vi "runner.vi"() -> ()   [LabVIEW 2010]
uses:
  common/xcontrols/XUserDropdown/XUserDropdown/XUserDropdown.xctl
  common/classes/ErrorController/ErrorController/ErrorController.lvclass
  <vilib>/Utility/miscctls.llb/LVPointTypeDef.ctl
  common/clusters/plugin_specification.ctl
  HelioWizardDL101109/wizard_cluster.ctl
  common/classes/GenericComponent/GenericComponent/GenericComponent.lvclass
  <vilib>/Platform/browser.llb/Open URL in Default Browser (string).vi
  common/classes/ErrorController/ErrorController/class_data.vi
panel:
  out "error loaded?":bool
  out "progress slider":i32(slide) scale=0.0..13.0
  in  "button: copy user":bool
  in  "button: delete user":bool
  in  "button: new user":bool
  in  "user":string(xcontrol)
  in  "mainConfigButton":bool
  in  "step":i32(listbox) caption="steps"
  in  "proceedButton":bool
  in  "backButton":bool
  in  "startButton":bool
  in  "wizard":string(combo) caption="Select a wizard"
  # "Wizard Runner"
  # "Procedure\n\n1. Select and start a wizard (it may take some time until all steps are loaded).\n\n2. Perform all configuration steps in the sequence given (note that there may be dependencies!).\n\n3. Edit main configuration.\n\nHint: Don't leave any component specifications empty in the configuration dialogs. Choose the generic version if a more specifiy component doesn't apply."
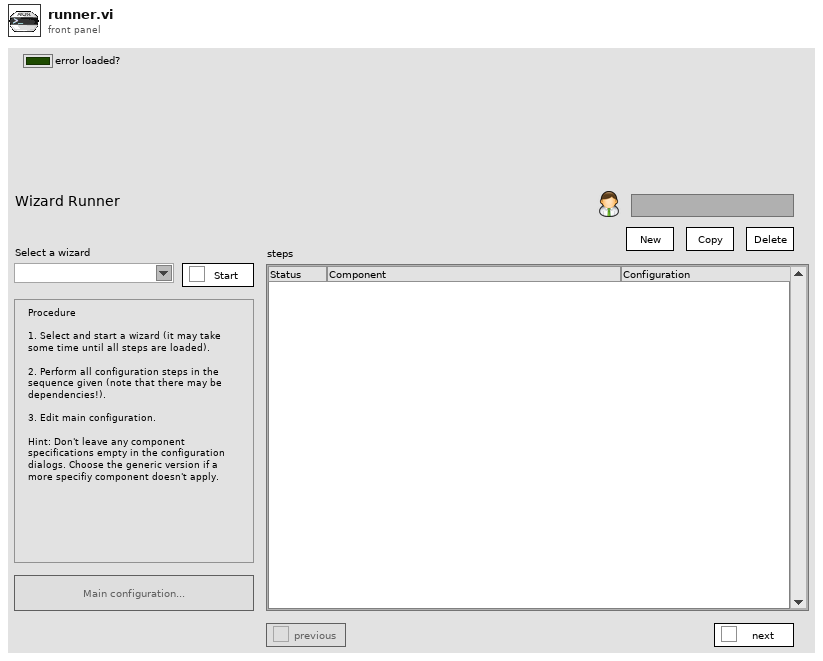
[diagram p1: front panel]
types:
  T1 = typedef "LVPointTypeDef.ctl" = cluster{"Horizontal":i16, "Vertical":i16}
  T2 = typedef "plugin_specification.ctl" = cluster{"class path":string, "configuration":string, "label":string, "settings name":string}
  T3 = typedef "wizard_cluster.ctl" = cluster{"step":T2[]}
  T4 = enum8{"Enabled", "Disabled", "Disabled and Grayed Out"}
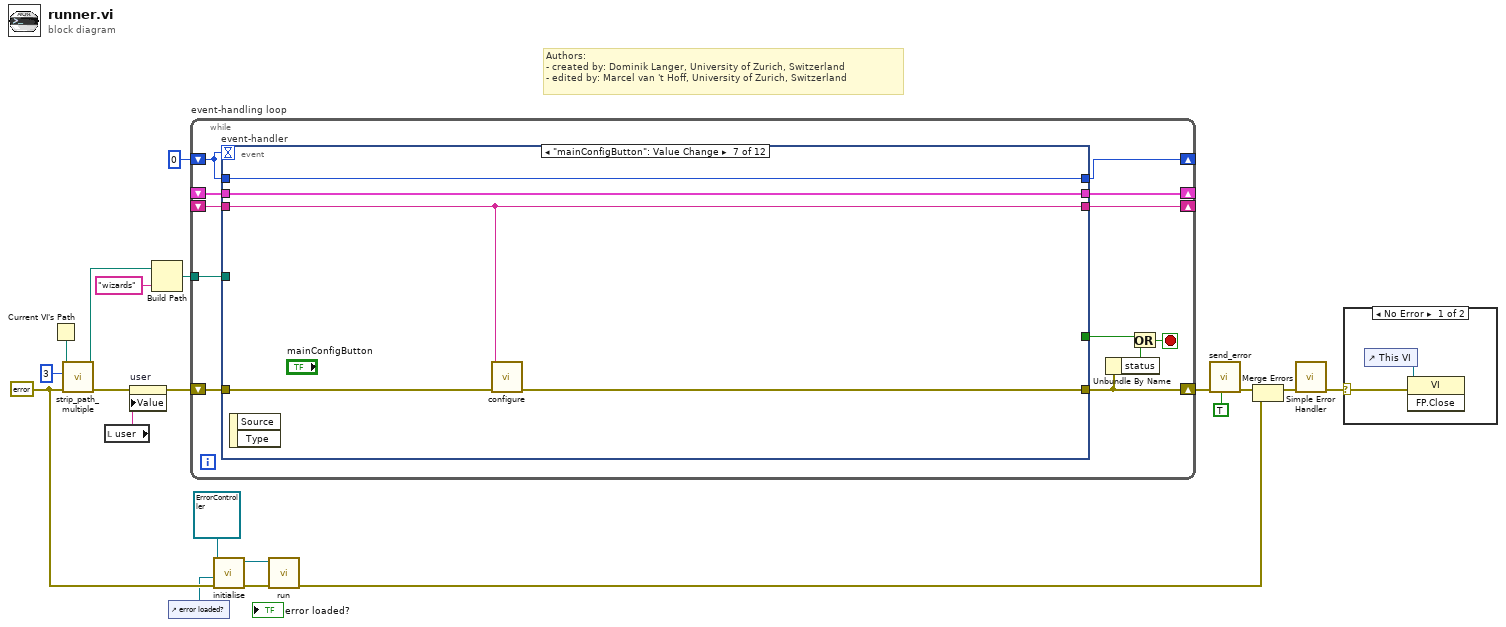
[diagram p0: block diagram]
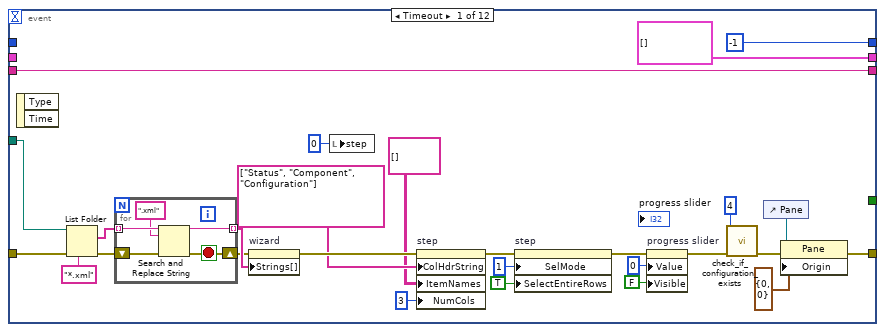
[diagram p3: hidden frame]
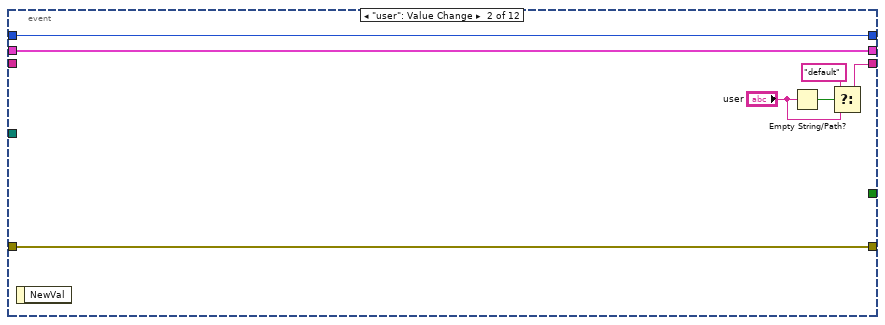
[diagram p4: hidden frame]
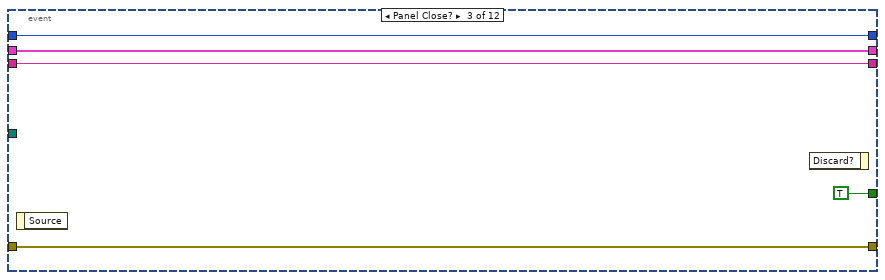
[diagram p5: hidden frame]
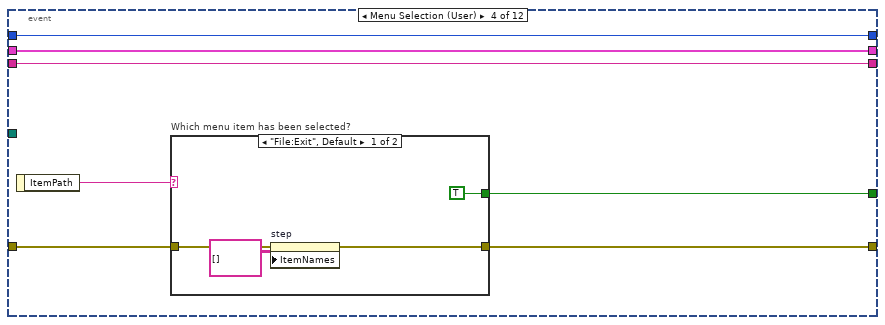
[diagram p6: hidden frame]
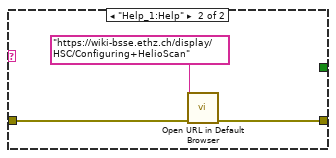
[diagram p7: hidden frame]
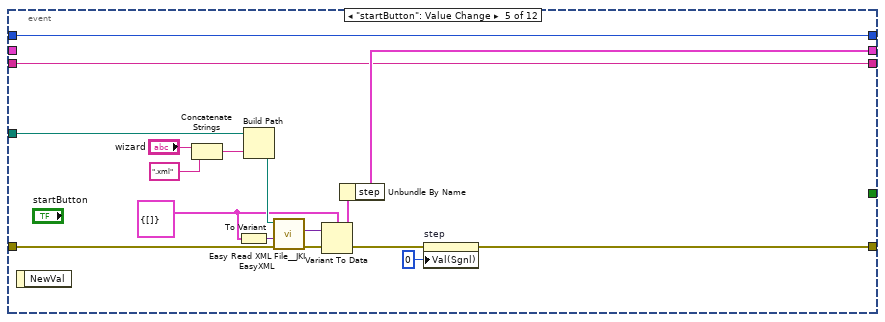
[diagram p8: hidden frame]
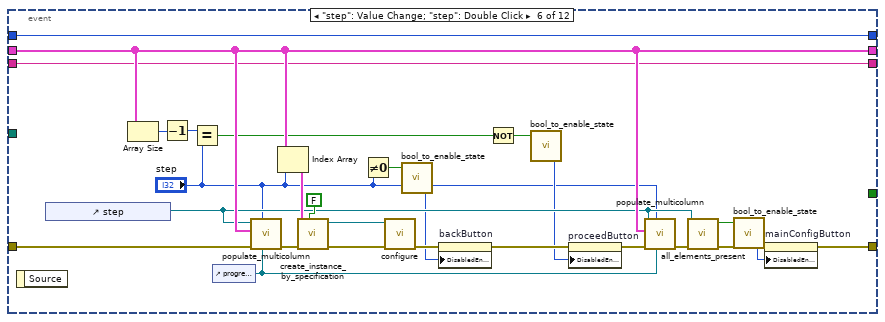
[diagram p9: hidden frame]
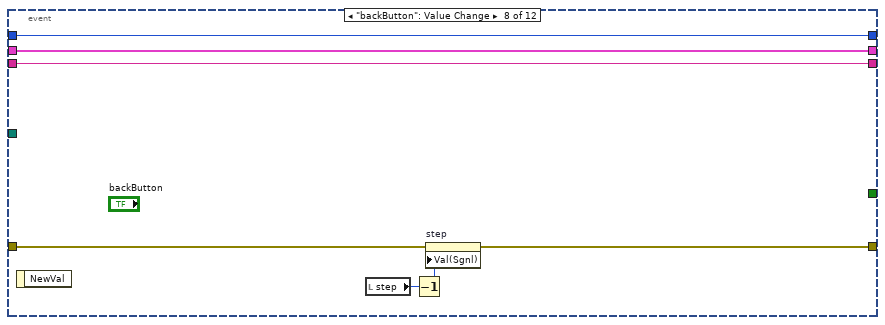
[diagram p10: hidden frame]
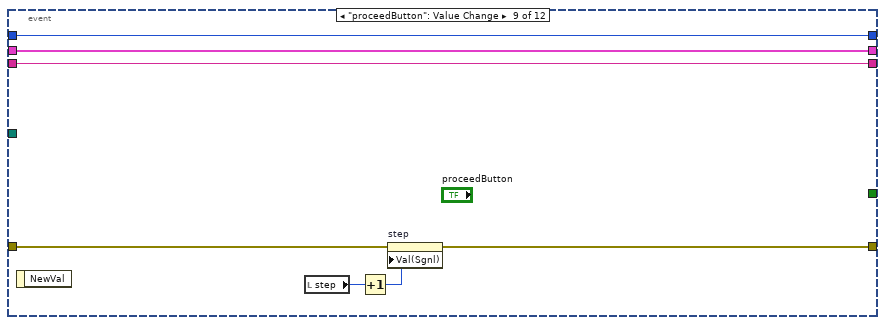
[diagram p11: hidden frame]
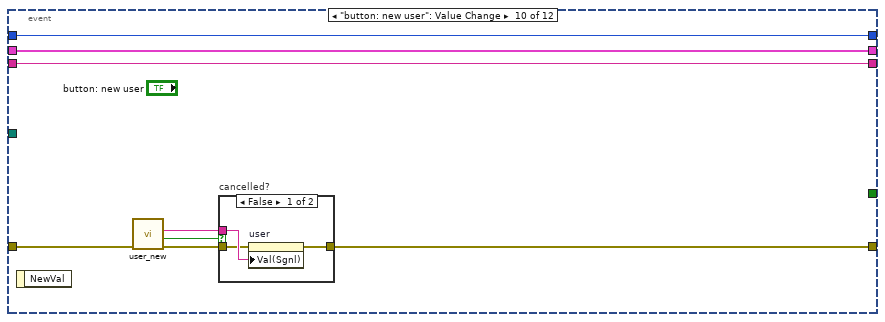
[diagram p12: hidden frame]
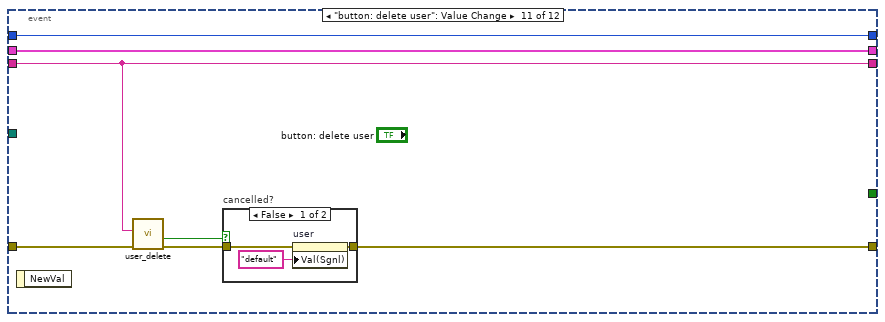
[diagram p14: hidden frame]
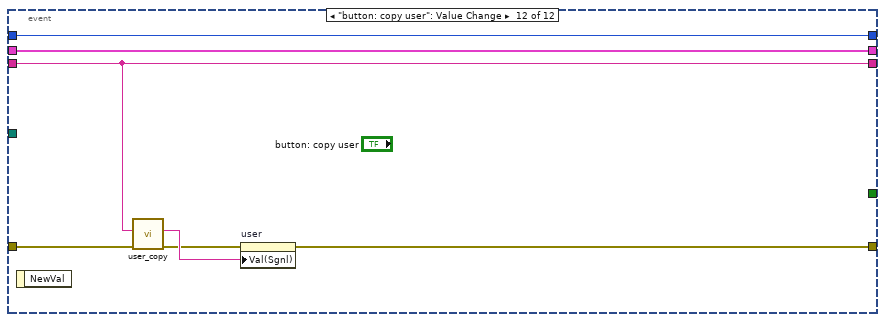
[diagram p16: hidden frame]
diagram:
  w5 = errorcluster {"status"=FALSE, "code"=0, "source"=""} ("error in (no error)")
  # "Authors: \n- created by: Dominik Langer, University of Zurich, Switzerland\n- edited by: Marcel van 't Hoff, University of Zurich, Switzerland"
  n1 = Current VI's Path() -> (path=w17:path)
  n2 = call "strip_path_multiple.vi"("error in (no error)"=w5, "number of strips"=3, "path in"=w17) -> ("error out"=w3:errorcluster, "path out"=w16:path)  [unwired: 7 in]
  n3 = local read "user"() -> (w1:string)
  n4 = property on="user" class="XUserDropdown (strict)"(error in=w3, "Value"=w1) -> (error out=w2:errorcluster)  [unwired: 1 in, 1 out]
  n5 = Build Path(base path=w16, name or relative path="wizards") -> (appended path=w18:path)
  n6 = control-ref of="error loaded?"() -> (w4:refnum<vi>)
  n7 = while "event-handling loop" {
    tunnel: w18 -> [w27]
    shift-right: [w25] -> _
    shift-left: _ -> [w26]
    shift-right: [w23] -> _
    shift-left: 0 -> [w24]
    shift-right: [w22] -> _
    shift-left: _ -> [w21]
    shift-right: [w31] -> w10
    shift-left: w2 -> [w32]
    stop <- w28 stop-if-true
    n8 = event "event-handler" shown="[6] \"mainConfigButton\": Value Change" {
      selector: _ -> [_ _ _ _ _ _ _ _ _ _ _ _]
      dyn-events: _ -> [_ _ _ _ _ _ _ _ _ _ _ _]
      timeout: w24 -> [_ _ _ _ _ _ _ _ _ _ _ _]
      tunnel: w32 -> [w56 w69 w76 w79 w107 w127 w137 w141 w149 w158 w170 w181]
      tunnel: [w35 w69 w76 w78 w95 w120 w136 w144 w148 w155 w167 w177] -> w31
      tunnel: [_ _ TRUE w80 _ _ _ _ _ _ _ _] -> w29
      tunnel: w27 -> [w57 _ _ _ w106 _ _ _ _ _ _ _]
      tunnel: [T2[] [] w71 w74 w83 w98 w124 w139 w146 w153 w161 w172 w183] -> w25
      tunnel: w26 -> [_ w71 w74 w83 _ w124 w139 w146 w153 w161 w172 w183]
      tunnel: [-1 w70 w73 w82 w101 w129 w138 w145 w152 w160 w171 w182] -> w23
      tunnel: w24 -> [_ w70 w73 w82 w101 w129 w138 w145 w152 w160 w171 w182]
      tunnel: [w46 w66 w72 w77 w94 w119 w135 w140 w147 w159 w169 w180] -> w22
      tunnel: w21 -> [w46 _ w72 w77 w94 w119 w135 w140 w147 w159 w169 w180]
      event Timeout {
        n9 = event-data() -> ()  [unwired: 1 in, 2 out]
        n10 = List Folder(path=w57, pattern="*.xml", error in=w56) -> (filenames=w40:string[], error out=w38:errorcluster)  [unwired: 1 in, 2 out]
        n11 = for {
          tunnel: w40 -> [w64] mode=indexing
          tunnel: [w62] -> w39 mode=indexing
          shift-right: [w60] -> w37
          shift-left: w38 -> [w61]
          stop <- w60 stop-if-true
          n12 = Search and Replace String(input string=w64, search string=".xml", error in=w61) -> (result string=w62:string, error out=w60:errorcluster)  [unwired: 5 in, 2 out]
        }
        n13 = property on="wizard" class="CmbBox"(error in=w37, "Strings[]"=w39) -> (error out=w54:errorcluster)  [unwired: 1 in, 1 out]
        n14 = local write "step"(0 ("step")) -> ()
        n15 = property on="step" class="MCListbox (strict)"(error in=w54, "ColHdrString"=string[] ["Status", "Component", "Configuration"] ("Item Names"), "ItemNames"=string[][] [] ("Item Names"), "NumCols"=u32 3 ("Number of Columns")) -> (error out=w48:errorcluster)  [unwired: 1 in, 1 out]
        n16 = property on="step" class="MCListbox (strict)"(error in=w48, "SelMode"=1 ("Selection Mode"), "SelectEntireRows"=TRUE ("Select Entire Rows")) -> (error out=w43:errorcluster)  [unwired: 1 in, 1 out]
        n17 = property on="progress slider" class="Slide (strict)"(error in=w43, "Value"=0 ("progress slider"), "Visible"=FALSE) -> (error out=w42:errorcluster)  [unwired: 1 in, 1 out]
        n18 = call "check_if_configuration_exists.vi"("error in (no error)"=w42, "number of strips"=4) -> ("error out"=w36:errorcluster)  [unwired: 9 in]
        n19 = control-ref of="Pane"() -> (w34:refnum<vi>)
        n20 = property class="Pane"(reference=w34, error in=w36, "Origin"=T1 {"Horizontal"=0, "Vertical"=0}) -> (error out=w35:errorcluster)  [unwired: 1 out]
      }
      event "user": Value Change {
        n21 = event-data() -> ()  [unwired: 1 in, 1 out]
        n22 = Empty String/Path?(string/path="user") -> (empty?=w68:bool)
        n23 = Select(t="default", s=w68, f="user") -> (s? t:f=w66:string)
      }
      event Panel Close? {
        n24 = event-data() -> ()  [unwired: 1 in, 1 out]
        n25 = event-data() -> ()  [unwired: 2 in, 1 out]
      }
      event Menu Selection (User) {
        n26 = event-data() -> ("ItemPath"=w81:string)  [unwired: 1 in]
        n27 = case "Which menu item has been selected?" shown="\"File:Exit\", Default" w81 {
          tunnel: [TRUE _] -> w80
          tunnel: w79 -> [w86 w90]
          tunnel: [w84 w89] -> w78
          frame "File:Exit", Default {
            n28 = property on="step" class="MCListbox (strict)"(error in=w86, "ItemNames"=string[][] [] ("Item Names")) -> (error out=w84:errorcluster)  [unwired: 1 in, 1 out]
          }
          frame "Help_1:Help" {
            n29 = call-poly <vilib>:"Open URL in Default Browser.vi"("error in (no error)"=w90, "URL"="https://wiki-bsse.ethz.ch/display/HSC/Configuring+HelioScan") -> ("error out"=w89:errorcluster)  [unwired: 4 in, 1 out]
          }
        }
      }
      event "startButton": Value Change {
        w99 = T3 {"step"=[]}
        n30 = event-data() -> ()  [unwired: 1 in, 1 out]
        n31 = Concatenate Strings("wizard", ".xml" ("string")) -> (w91:string)
        n32 = To Variant(anything=w99) -> (Variant=w104:variant)
        n33 = Build Path(base path=w106, name or relative path=w91) -> (appended path=w105:path)
        n34 = call <vilib>:"Easy Read XML File__JKI EasyXML.vi"("error in (no error)"=w107, "LabVIEW Data (Type)"=w104, "XML File Path"=w105) -> ("error out"=w103:errorcluster, "LabVIEW Data"=w102:variant)  [unwired: 6 in, 1 out]
        n35 = Variant To Data(error in=w103, Variant=w102, type=w99) -> (error out=w96:errorcluster, data=w100:T3)
        n36 = Unbundle By Name(w100) -> ("step"=w98:T2[])
        n37 = property on="step" class="MCListbox (strict)"(error in=w96, "Val(Sgnl)"=0 ("Value (Signaling)")) -> (error out=w95:errorcluster)  [unwired: 1 in, 1 out]
      }
      event "step": Value Change; "step": Double Click {
        n38 = event-data() -> ()  [unwired: 1 in, 1 out]
        n39 = control-ref of="step"() -> (w122:refnum<vi>)
        n40 = Array Size(array=w124) -> (size(s)=w131:i32)
        n41 = Decrement(x=w131) -> (x-1=w130:i32)
        n42 = Equal?(x=w130, y="step") -> (x = y?=w113:bool)
        n43 = control-ref of="progress slider"() -> (w118:refnum<vi>)
        n44 = call "populate_multicolumn.vi"("progress slider"=w118, "selected item (index)"="step", "error in (no error)"=w127, "steps"=w124, "multicolumn list box"=w122) -> ("error out"=w126:errorcluster)  [unwired: 6 in]
        n45 = Index Array(array=w124, index="step") -> (element=w134:T2)
        n46 = call "create_instance_by_specification.vi"("call constructor?"=FALSE, "error in (no error)"=w126, "component specification"=w134) -> ("error out"=w116:errorcluster, "GenericPlugin out"=w117:refnum<class "GenericComponent.lvclass">)  [unwired: 6 in, 1 out]
        n47 = Not Equal To 0?(x="step") -> (x != 0?=w109:bool)
        n48 = call-dynamic "configure.vi"("error in (no error)"=w116, "GenericPlugin in"=w117) -> ("error out"=w133:errorcluster)  [unwired: 8 in, 1 out]
        n49 = call "bool_to_enable_state.vi"("boolean in"=w109) -> ("enabled status out"=w110:T4)  [unwired: 4 in]
        n50 = property on="backButton" class="Bool"(error in=w133, "DisabledEnum"=w110) -> (error out=w132:errorcluster)  [unwired: 1 in, 1 out]
        n51 = Not(x=w113) -> (.not. x?=w111:bool)
        n52 = call "bool_to_enable_state.vi"("boolean in"=w111) -> ("enabled status out"=w112:T4)  [unwired: 4 in]
        n53 = property on="proceedButton" class="Bool"(error in=w132, "DisabledEnum"=w112) -> (error out=w125:errorcluster)  [unwired: 1 in, 1 out]
        n54 = call "populate_multicolumn.vi"("progress slider"=w118, "selected item (index)"="step", "error in (no error)"=w125, "steps"=w124, "multicolumn list box"=w122) -> ("error out"=w123:errorcluster)  [unwired: 6 in]
        n55 = call "all_elements_present.vi"("error in (no error)"=w123, "multicolumn list box"=w122) -> ("error out"=w121:errorcluster, "all elements are present"=w115:bool)  [unwired: 8 in]
        n56 = call "bool_to_enable_state.vi"("boolean in"=w115) -> ("enabled status out"=w114:T4)  [unwired: 4 in]
        n57 = property on="mainConfigButton" class="Bool"(error in=w121, "DisabledEnum"=w114) -> (error out=w120:errorcluster)  [unwired: 1 in, 1 out]
      }
      event "mainConfigButton": Value Change {
        n58 = event-data() -> ()  [unwired: 1 in, 2 out]
        n59 = call "configure.vi"("error in (no error)"=w137, "user"=w135) -> ("error out"=w136:errorcluster)  [unwired: 8 in, 1 out]
      }
      event "backButton": Value Change {
        n60 = event-data() -> ()  [unwired: 1 in, 1 out]
        n61 = local read "step"() -> (w142:i32)
        n62 = Decrement(x=w142) -> (x-1=w143:i32)
        n63 = property on="step" class="MCListbox (strict)"(error in=w141, "Val(Sgnl)"=w143) -> (error out=w144:errorcluster)  [unwired: 1 in, 1 out]
      }
      event "proceedButton": Value Change {
        n64 = event-data() -> ()  [unwired: 1 in, 1 out]
        n65 = local read "step"() -> (w151:i32)
        n66 = Increment(x=w151) -> (x+1=w150:i32)
        n67 = property on="step" class="MCListbox (strict)"(error in=w149, "Val(Sgnl)"=w150) -> (error out=w148:errorcluster)  [unwired: 1 in, 1 out]
      }
      event "button: new user": Value Change {
        n68 = event-data() -> ()  [unwired: 1 in, 1 out]
        n69 = call "user_new.vi"("error in (no error)"=w158) -> ("error IO"=w156:errorcluster, "cancelled?"=w154:bool, "user name out"=w157:string)  [unwired: 8 in]
        n70 = case "cancelled?" shown="False" w154 {
          tunnel: w157 -> [w164 _]
          tunnel: w156 -> [w163 w165]
          tunnel: [w162 w165] -> w155
          frame False {
            n71 = property on="user" class="XUserDropdown (strict)"(error in=w163, "Val(Sgnl)"=w164) -> (error out=w162:errorcluster)  [unwired: 1 in, 1 out]
          }
          frame True {
          }
        }
      }
      event "button: delete user": Value Change {
        n72 = event-data() -> ()  [unwired: 1 in, 1 out]
        n73 = call "user_delete.vi"("error in (no error)"=w170, "user name in"=w169) -> ("error out"=w168:errorcluster, "cancelled?"=w166:bool)  [unwired: 8 in]
        n74 = case "cancelled?" shown="False" w166 {
          tunnel: w168 -> [w174 w176]
          tunnel: [w173 w176] -> w167
          frame False {
            n75 = property on="user" class="XUserDropdown (strict)"(error in=w174, "Val(Sgnl)"="default" ("Value (Signaling)")) -> (error out=w173:errorcluster)  [unwired: 1 in, 1 out]
          }
          frame True {
          }
        }
      }
      event "button: copy user": Value Change {
        n76 = event-data() -> ()  [unwired: 1 in, 1 out]
        n77 = call "user_copy.vi"("error in (no error)"=w181, "old user name in"=w180) -> ("error out"=w178:errorcluster, "new user name out"=w179:string)  [unwired: 7 in, 1 out]
        n78 = property on="user" class="XUserDropdown (strict)"(error in=w178, "Val(Sgnl)"=w179) -> (error out=w177:errorcluster)  [unwired: 1 in, 1 out]
      }
    }
    n79 = Unbundle By Name(w31) -> ("status"=w30:bool)
    n80 = Or(x=w29, y=w30) -> (x .or. y?=w28:bool)
  }
  n81 = call-dynamic "initialise.vi"("error in (no error)"=w5, "error boolean"=w4, "ErrorController in"=refnum<class "ErrorController.lvclass"> refnum) -> ("error out"=w12:errorcluster, "ErrorController out"=w11:refnum<class "ErrorController.lvclass">)  [unwired: 7 in]
  n82 = call "run.vi"("error in (no error)"=w12, "ErrorController in"=w11) -> ("error out"=w8:errorcluster)  [unwired: 8 in, 1 out]
  n83 = call "send_error.vi"("last error? (F)"=TRUE, "error in (no error)"=w10) -> ("error out"=w7:errorcluster)  [unwired: 9 in]
  n84 = Merge Errors(w7, w8) -> (w6:errorcluster)
  n85 = call <vilib>:"Simple Error Handler.vi"("error in (no error)"=w6) -> ("error out"=w14:errorcluster)  [unwired: 4 in, 4 out]
  n86 = case shown="No Error" w14 {
    selector: w14 -> [w185 _]
    frame No Error {
      n87 = control-ref of="This VI"() -> (w184:refnum<vi>)
      n88 = invoke class="VI" method="FP.Close"(reference=w184, error in=w185) -> ()  [unwired: 1 in, 3 out]
    }
    frame Error {
    }
  }
